vi "Cursors2Freq.vi"(0 "Cursor 1 eV":dbl, 1 "Cursor 2 eV":dbl) -> (2 "Cursor dE":dbl, 3 "Cursor 1 nm":dbl, 4 "Cursor 2 nm":dbl, 5 "Cursor dnm":dbl)   [LabVIEW 2019]
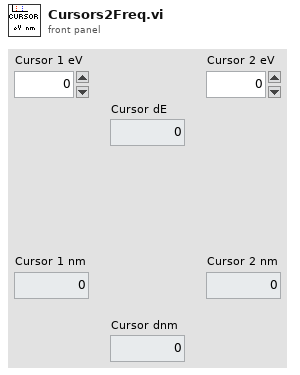
[diagram p1: front panel]
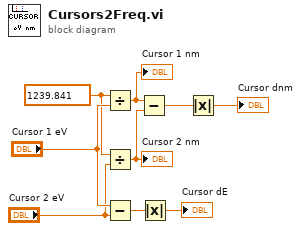
[diagram p0: block diagram]
diagram:
  w1 = 1239.841
  n1 = Divide(x=w1, y="Cursor 1 eV") -> (x/y=w6:dbl)
  "Cursor 1 nm" <- w6
  n2 = Divide(x=w1, y="Cursor 2 eV") -> (x/y=w5:dbl)
  "Cursor 2 nm" <- w5
  n3 = Subtract(x="Cursor 1 eV", y="Cursor 2 eV") -> (x-y=w9:dbl)
  n4 = Subtract(x=w6, y=w5) -> (x-y=w4:dbl)
  n5 = Absolute Value(x=w9) -> (abs(x)=→"Cursor dE":dbl)
  n6 = Absolute Value(x=w4) -> (abs(x)=→"Cursor dnm":dbl)
